vi "Parse inputs.vi"(10 "Inputs":string[](array[string]), 11 "PrintToSingleFileHtml in":refnum<class "PrintToSingleFileHtml.lvclass">) -> (3 "PrintToSingleFileHtml out":refnum<class "PrintToSingleFileHtml.lvclass">)   [LabVIEW 2026, in "PrintToSingleFileHtml.lvclass"]
uses:
  PrintToSingleFileHtml.lvclass
  PrintToSingleFileHtml.lvclass/PrintToSingleFileHtml.ctl
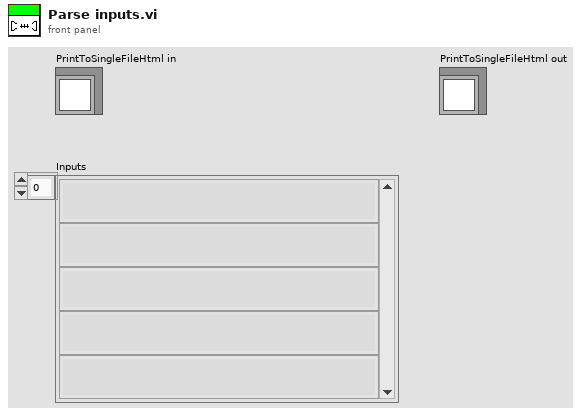
[diagram p1: front panel]
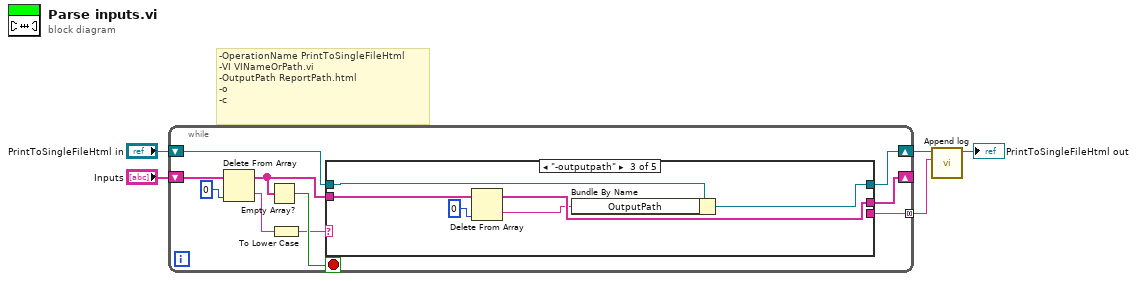
[diagram p0: block diagram]
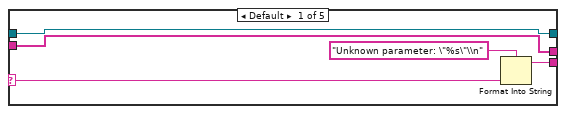
[diagram p2: hidden frame]
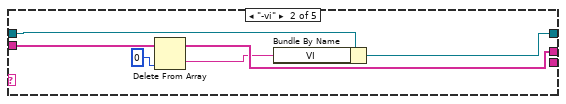
[diagram p3: hidden frame]
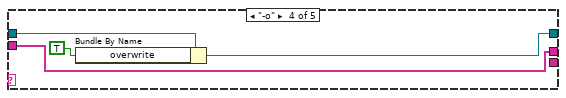
[diagram p4: hidden frame]
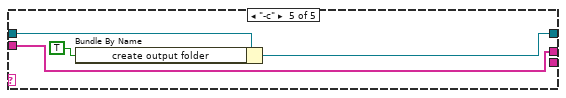
[diagram p5: hidden frame]
diagram:
  # "-OperationName PrintToSingleFileHtml\n-VI VINameOrPath.vi\n-OutputPath ReportPath.html\n-o\n-c"
  n1 = while {
    shift-right: [w12] -> _
    shift-left: "Inputs" -> [w15]
    shift-right: [w10] -> w3
    shift-left: "PrintToSingleFileHtml in" -> [w11]
    tunnel: [w7] -> w1 mode=concatenating
    stop <- w8 stop-if-true
    n2 = Delete From Array(array=w15, index=0) -> (deleted portion=w13:string, array with subset deleted=w9:string[])  [unwired: 1 in]
    n3 = Empty Array?(array=w9) -> (empty?=w8:bool)
    n4 = To Lower Case(string=w13) -> (all lower case string=w6:string)
    n5 = case shown="\"-outputpath\"" w6 {
      selector: w6 -> [w18 _ _ _ _]
      tunnel: [w20 w24 w30 w36 w40] -> w12
      tunnel: w9 -> [w20 w25 w31 w36 w40]
      tunnel: w11 -> [w19 w23 w29 w35 w39]
      tunnel: [w19 w22 w28 w34 w38] -> w10
      tunnel: [w16 _ _ _ _] -> w7
      frame Default {
        n6 = Format Into String(format string="Unknown parameter: \"%s\"\\n", w18) -> (resulting string=w16:string)  [unwired: 2 in, 1 out]
      }
      frame "-vi" {
        n7 = Delete From Array(array=w25, index=0) -> (deleted portion=w21:string, array with subset deleted=w24:string[])  [unwired: 1 in]
        n8 = Bundle By Name(cluster=w23, "VI"=w21) -> (w22:refnum<class "PrintToSingleFileHtml.lvclass">)
      }
      frame "-outputpath" {
        n9 = Delete From Array(array=w31, index=0) -> (deleted portion=w27:string, array with subset deleted=w30:string[])  [unwired: 1 in]
        n10 = Bundle By Name(cluster=w29, "OutputPath"=w27) -> (w28:refnum<class "PrintToSingleFileHtml.lvclass">)
      }
      frame "-o" {
        n11 = Bundle By Name(cluster=w35, "overwrite"=TRUE ("parameters.overwrite")) -> (w34:refnum<class "PrintToSingleFileHtml.lvclass">)
      }
      frame "-c" {
        n12 = Bundle By Name(cluster=w39, "create output folder"=TRUE ("parameters.overwrite")) -> (w38:refnum<class "PrintToSingleFileHtml.lvclass">)
      }
    }
  }
  n13 = call "Append log.vi"("message"=w1, "PrintToSingleFileHtml in"=w3) -> ("PrintToSingleFileHtml out"=→"PrintToSingleFileHtml out":refnum<class "PrintToSingleFileHtml.lvclass">)  [unwired: 9 in]
